vi "CNT Material Properties.vi"(6 "m-nm CNT":dbl, 9 "CNT Thickness (CNT Length)":dbl, 10 "Energy (Heat; I^2R)":dbl, 11 "NS Base Area":dbl) -> (1 "Mass CNTs":dbl, 2 "Delta Temp Change CNT":dbl, 3 "CNT Specfic Heat Capacity":dbl, 4 "CNT Density":dbl, 5 "Volume CNT":dbl, 7 "CNT Thickness":dbl, 8 "mc":dbl)   [LabVIEW 2020]
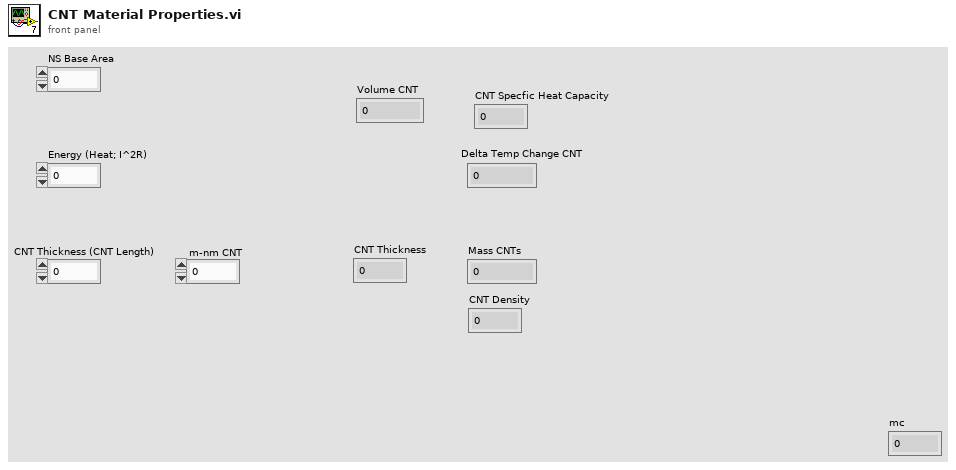
[diagram p1: front panel]
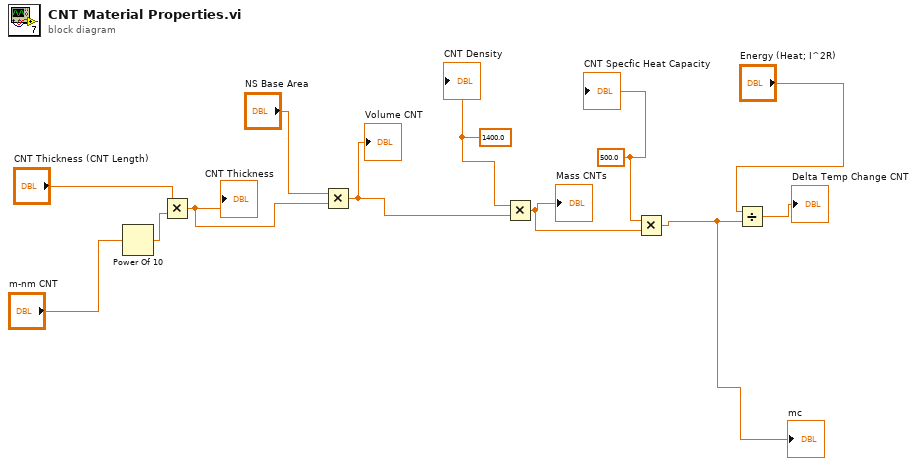
[diagram p0: block diagram]
diagram:
  w12 = 500.0 ("Silicon Specfic Heat Capacity 7")
  w6 = 1400.0 ("Silicon Density 7")
  n1 = Power Of 10(x="m-nm CNT") -> (10^x=w2:dbl)
  n2 = Multiply(x="CNT Thickness (CNT Length)", y=w2) -> (x*y=w5:dbl)
  "CNT Thickness" <- w5
  n3 = Multiply(x="NS Base Area", y=w5) -> (x*y=w7:dbl)
  "Volume CNT" <- w7
  n4 = Multiply(x=w6, y=w7) -> (x*y=w11:dbl)
  "Mass CNTs" <- w11
  n5 = Multiply(x=w12, y=w11) -> (x*y=w1:dbl)
  "mc" <- w1
  n6 = Divide(x="Energy (Heat; I^2R)", y=w1) -> (x/y=→"Delta Temp Change CNT":dbl)
  "CNT Density" <- w6
  "CNT Specfic Heat Capacity" <- w12
